vi "Parse Timezone.vi"(8 "error in (no error)":errorcluster, 11 "Timezone String":string) -> (0 "error out":errorcluster, 3 "time zone offset":T1)   [LabVIEW 2013, in "JKI JSON Serialization.lvlib" / "JSON Deserializer.lvclass"]
doc: "JKI Serialization 1.0.0.4\nTomi Maila - JKI\nCopyright (c) 2016, JKI"
uses:
  JSON Deserializer.lvclass
  <vilib>/regexp/Match Regular Expression.xnode
  <vilib>/Utility/miscctls.llb/LVDateTimeRec.ctl
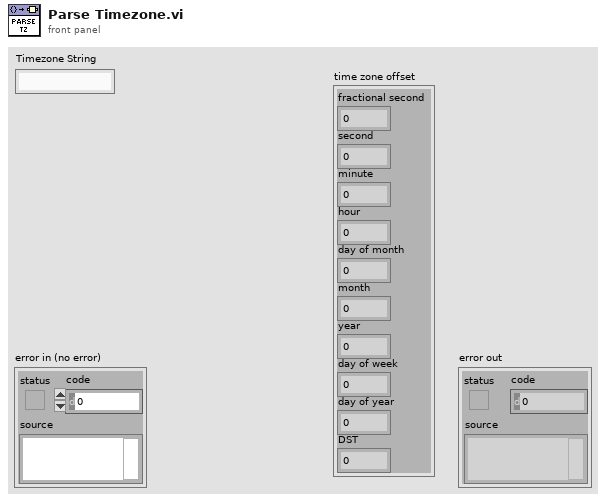
[diagram p1: front panel]
types:
  T1 = typedef "LVDateTimeRec.ctl" = cluster{"fractional second":dbl, "second":i32, "minute":i32, "hour":i32, "day of month":i32, "month":i32, "year":i32, "day of week":i32, "day of year":i32, "DST":i32}
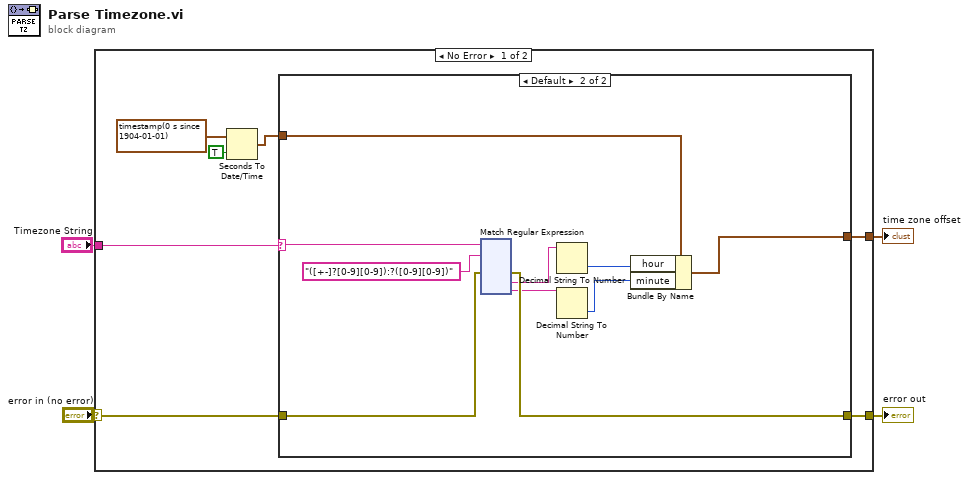
[diagram p0: block diagram]
diagram:
  n1 = case shown="No Error" "error in (no error)" {
    selector: "error in (no error)" -> [w10 w141]
    tunnel: [w9 w141] -> w3
    tunnel: "Timezone String" -> [w11 _]
    tunnel: [w8 _] -> w1
    frame No Error {
      n2 = Seconds To Date/Time(time stamp (now)=timestamp(0 s since 1904-01-01), to UTC (F)=TRUE) -> (date time rec=w6:T1)
      n3 = case shown="Default" w11 {
        selector: w11 -> [_ w23]
        tunnel: w10 -> [w13 w21]
        tunnel: [w13 w20] -> w9
        tunnel: [w12 w14] -> w8
        tunnel: w6 -> [w12 w17]
        frame "Z", "z" {
        }
        frame Default {
          n4 = xnode "Match Regular Expression"("input string"=w23, "regular expression"="([+-]?[0-9][0-9]):?([0-9][0-9])", "error in"=w21) -> ("error out"=w20:errorcluster, "submatch 1"=w19:string, "submatch 2"=w18:string)  [unwired: 3 in, 4 out]
          n5 = Decimal String To Number(string=w19) -> (number=w16:i32)  [unwired: 2 in, 1 out]
          n6 = Decimal String To Number(string=w18) -> (number=w15:i32)  [unwired: 2 in, 1 out]
          n7 = Bundle By Name(cluster=w17, "hour"=w16, "minute"=w15) -> (w14:T1)
        }
      }
    }
    frame Error {
    }
  }
  "error out" <- w3
  "time zone offset" <- w1
